vi "Read Calibrations+Settings.vi"   [LabVIEW 2014]
uses:
  Global Variables/Calibrations.vi
  Global Variables/Settings.vi
types:
  T1 = cluster{"proportional gain (Kc)":dbl, "integral time (Ti, min)":dbl, "derivative time (Td, min)":dbl, "Maximum Value":dbl, "Minimum Value":dbl, "epsilon":dbl}
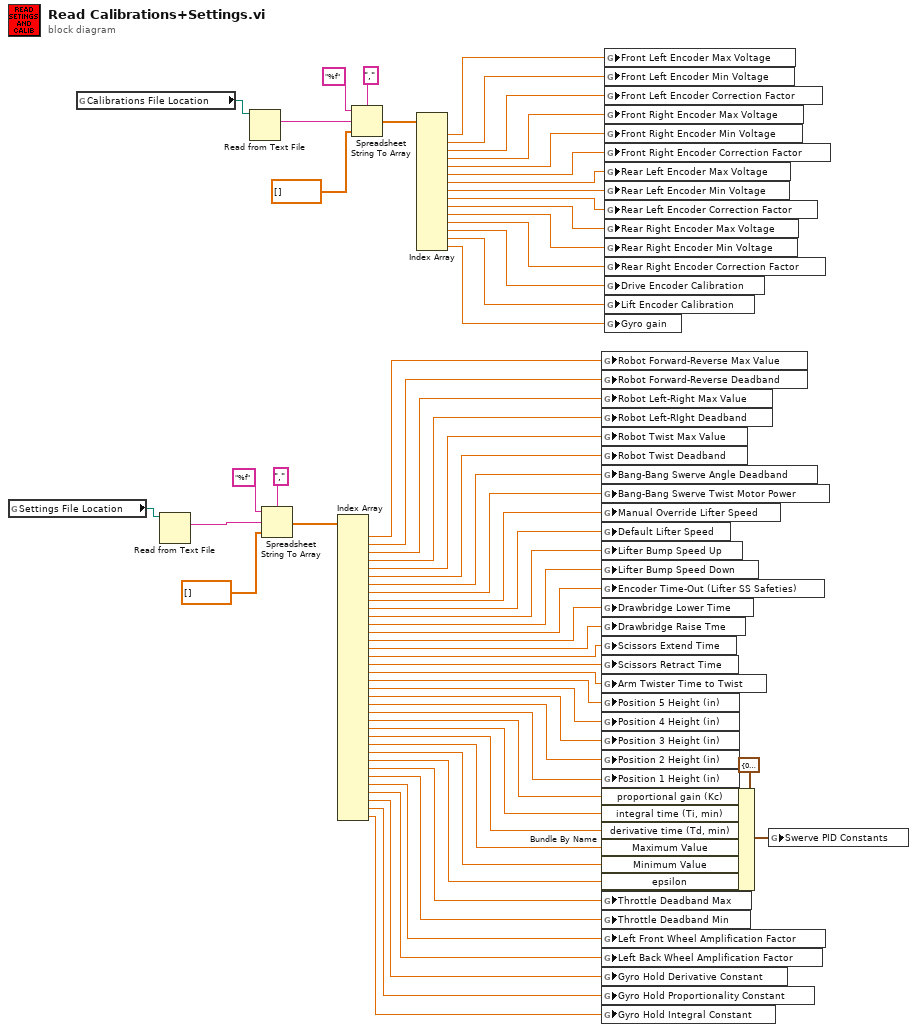
[diagram p0: block diagram]
diagram:
  n1 = global read "Settings.vi" "Settings File Location"() -> (w40:path)
  n2 = global read "Calibrations.vi" "Calibrations File Location"() -> (w61:path)
  n3 = Read from Text File(file (use dialog)=w40) -> (text=w41:string)  [unwired: 3 in, 3 out]
  n4 = Read from Text File(file (use dialog)=w61) -> (text=w65:string)  [unwired: 3 in, 3 out]
  n5 = Spreadsheet String To Array(delimiter (Tab)=",", format string="%f", spreadsheet string=w41, array type (2D Dbl)=dbl[] []) -> (array=w4:dbl[])
  n6 = Index Array(array=w4) -> (element #1=w11:dbl, element #2=w10:dbl, element #3=w37:dbl, element #4=w36:dbl, element #5=w35:dbl, element #6=w34:dbl, element #7=w33:dbl, element #8=w32:dbl, element #9=w31:dbl, element #10=w30:dbl, element #11=w29:dbl, element #12=w28:dbl, element #13=w27:dbl, element #14=w26:dbl, element #15=w25:dbl, element #16=w24:dbl, element #17=w23:dbl, element #18=w12:dbl, element #19=w22:dbl, element #20=w21:dbl, element #21=w20:dbl, element #22=w19:dbl, element #23=w18:dbl, element #24=w17:dbl, element #25=w9:dbl, element #26=w16:dbl, element #27=w15:dbl, element #28=w14:dbl, element #29=w13:dbl, element #30=w8:dbl, element #31=w7:dbl, element #32=w6:dbl, element #33=w5:dbl, element #34=w3:dbl, element #35=w2:dbl, element #36=w1:dbl)  [unwired: 36 in]
  n7 = Spreadsheet String To Array(delimiter (Tab)=",", format string="%f", spreadsheet string=w65, array type (2D Dbl)=dbl[] []) -> (array=w60:dbl[])
  n8 = Index Array(array=w60) -> (element #1=w59:dbl, element #2=w58:dbl, element #3=w57:dbl, element #4=w56:dbl, element #5=w55:dbl, element #6=w54:dbl, element #7=w53:dbl, element #8=w52:dbl, element #9=w51:dbl, element #10=w45:dbl, element #11=w50:dbl, element #12=w49:dbl, element #13=w47:dbl, element #14=w48:dbl, element #15=w46:dbl)  [unwired: 15 in]
  n9 = global write "Settings.vi" "Robot Forward-Reverse Max Value"(w11) -> ()
  n10 = global write "Settings.vi" "Robot Forward-Reverse Deadband"(w10) -> ()
  n11 = global write "Settings.vi" "Robot Left-Right Max Value"(w37) -> ()
  n12 = global write "Settings.vi" "Robot Left-RIght Deadband"(w36) -> ()
  n13 = global write "Settings.vi" "Robot Twist Max Value"(w35) -> ()
  n14 = global write "Settings.vi" "Robot Twist Deadband"(w34) -> ()
  n15 = global write "Settings.vi" "Bang-Bang Swerve Angle Deadband"(w33) -> ()
  n16 = global write "Settings.vi" "Bang-Bang Swerve Twist Motor Power"(w32) -> ()
  n17 = global write "Settings.vi" "Manual Override Lifter Speed"(w31) -> ()
  n18 = global write "Settings.vi" "Default Lifter Speed"(w30) -> ()
  n19 = global write "Settings.vi" "Lifter Bump Speed Up"(w29) -> ()
  n20 = global write "Settings.vi" "Lifter Bump Speed Down"(w28) -> ()
  n21 = global write "Settings.vi" "Encoder Time-Out (Lifter SS Safeties)"(w27) -> ()
  n22 = global write "Settings.vi" "Drawbridge Lower Time"(w26) -> ()
  n23 = global write "Settings.vi" "Drawbridge Raise Tme"(w25) -> ()
  n24 = global write "Settings.vi" "Scissors Extend Time"(w24) -> ()
  n25 = global write "Settings.vi" "Scissors Retract Time"(w23) -> ()
  n26 = global write "Settings.vi" "Arm Twister Time to Twist"(w12) -> ()
  n27 = global write "Settings.vi" "Position 5 Height (in)"(w22) -> ()
  n28 = global write "Settings.vi" "Position 4 Height (in)"(w21) -> ()
  n29 = global write "Settings.vi" "Position 3 Height (in)"(w20) -> ()
  n30 = global write "Settings.vi" "Position 2 Height (in)"(w19) -> ()
  n31 = global write "Settings.vi" "Position 1 Height (in)"(w18) -> ()
  n32 = Bundle By Name(cluster=T1 {"proportional gain (Kc)"=0.025, "integral time (Ti, min)"=0.0, "derivative time (Td, min)"=0.0005, "Maximum Value"=0.0005, "Minimum Value"=0.0005, "epsilon"=0.0005} ("Swerve PID Constants"), "proportional gain (Kc)"=w17, "integral time (Ti, min)"=w9, "derivative time (Td, min)"=w16, "Maximum Value"=w15, "Minimum Value"=w14, "epsilon"=w13) -> (w39:T1)
  n33 = global write "Settings.vi" "Throttle Deadband Max"(w8) -> ()
  n34 = global write "Settings.vi" "Throttle Deadband Min"(w7) -> ()
  n35 = global write "Settings.vi" "Left Front Wheel Amplification Factor"(w6) -> ()
  n36 = global write "Settings.vi" "Left Back Wheel Amplification Factor"(w5) -> ()
  n37 = global write "Settings.vi" "Gyro Hold Derivative Constant"(w3) -> ()
  n38 = global write "Settings.vi" "Gyro Hold Proportionality Constant"(w2) -> ()
  n39 = global write "Settings.vi" "Gyro Hold Integral Constant"(w1) -> ()
  n40 = global write "Calibrations.vi" "Front Left Encoder Max Voltage"(w59) -> ()
  n41 = global write "Calibrations.vi" "Front Left Encoder Min Voltage"(w58) -> ()
  n42 = global write "Calibrations.vi" "Front Left Encoder Correction Factor"(w57) -> ()
  n43 = global write "Calibrations.vi" "Front Right Encoder Max Voltage"(w56) -> ()
  n44 = global write "Calibrations.vi" "Front Right Encoder Min Voltage"(w55) -> ()
  n45 = global write "Calibrations.vi" "Front Right Encoder Correction Factor"(w54) -> ()
  n46 = global write "Calibrations.vi" "Rear Left Encoder Max Voltage"(w53) -> ()
  n47 = global write "Calibrations.vi" "Rear Left Encoder Min Voltage"(w52) -> ()
  n48 = global write "Calibrations.vi" "Rear Left Encoder Correction Factor"(w51) -> ()
  n49 = global write "Calibrations.vi" "Rear Right Encoder Max Voltage"(w45) -> ()
  n50 = global write "Calibrations.vi" "Rear Right Encoder Min Voltage"(w50) -> ()
  n51 = global write "Calibrations.vi" "Rear Right Encoder Correction Factor"(w49) -> ()
  n52 = global write "Calibrations.vi" "Drive Encoder Calibration"(w47) -> ()
  n53 = global write "Calibrations.vi" "Lift Encoder Calibration"(w48) -> ()
  n54 = global write "Calibrations.vi" "Gyro gain"(w46) -> ()
  n55 = global write "Settings.vi" "Swerve PID Constants"(w39) -> ()
